vi "Define Channel Count.vi"(8 "error in":errorcluster, 11 "NI 9482 in":refnum<class "NI 9482.lvclass">) -> (0 "error out":errorcluster, 3 "NI 9482 out":refnum<class "NI 9482.lvclass">)   [LabVIEW 2017, in "Scan Engine Scripting.lvlib" / "NI 9482.lvclass"]
uses:
  NI 9482.lvclass
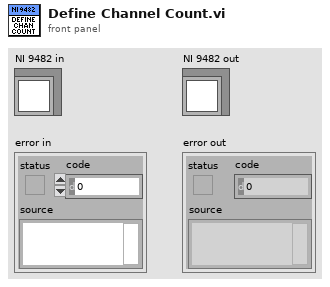
[diagram p1: front panel]
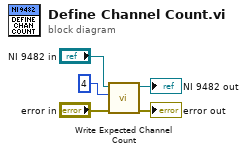
[diagram p0: block diagram]
diagram:
  n1 = call-dynamic "Write Expected Channel Count.vi"("error in"="error in", "expected channel count"=4, "module in"="NI 9482 in") -> ("error out"=→"error out":errorcluster, "module out"=→"NI 9482 out":refnum<class "NI 9482.lvclass">)  [unwired: 7 in]
